vi "read_matrices.vi"() -> (0 "Matrix Matlab":T1, 1 "Trajectory":T1)   [LabVIEW 2021]
uses:
  <vilib>/Analysis/Matrix/Datatypes/RealMatrix.ctl
  <vilib>/Utility/file.llb/Read Delimited Spreadsheet (DBL).vi
  <vilib>/Analysis/Matrix/NI_Matrix.lvlib
panel:
  out "error out 2":errorcluster
  in  "delimiter (,) 2":string=","
  in  "error in (no error) 2":errorcluster
  in  "file path (dialog if empty) 2":path=path "c:/ni-rt/startup/trajectorymat.csv"
  out "error out":errorcluster
  in  "delimiter (,)":string=","
  in  "error in (no error)":errorcluster
  in  "file path (dialog if empty)":path=path "c:/ni-rt/startup/matrixmat.csv"
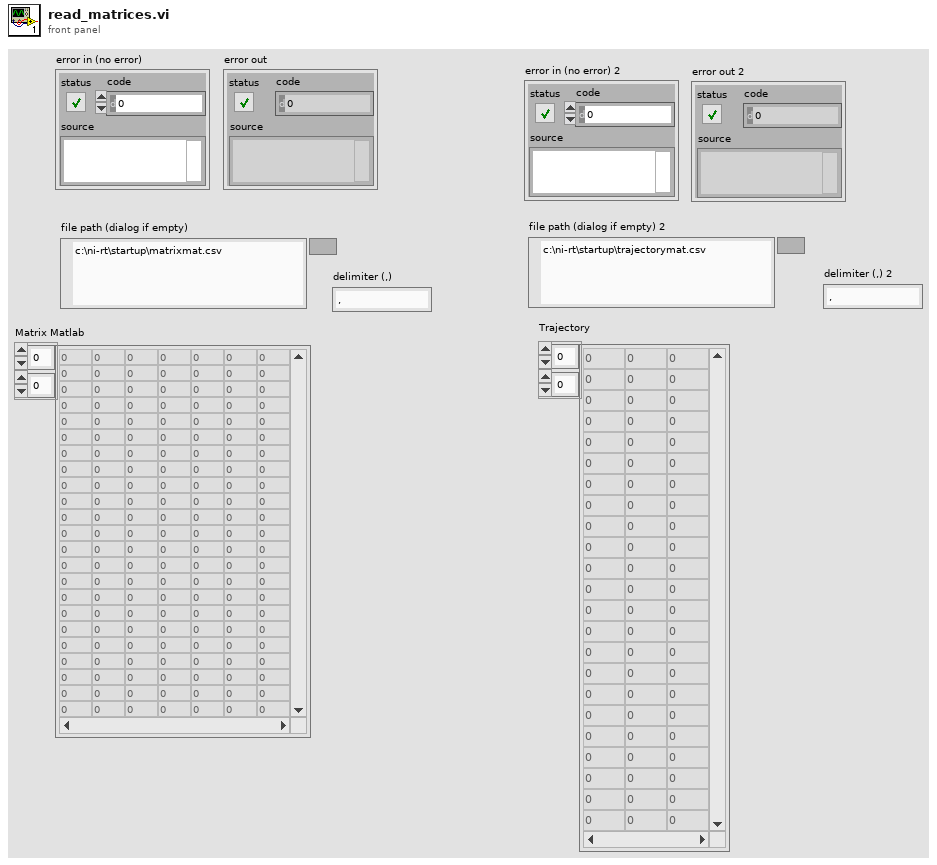
[diagram p1: front panel]
types:
  T1 = typedef "NI_Matrix.lvlib/RealMatrix.ctl" = dbl[][]
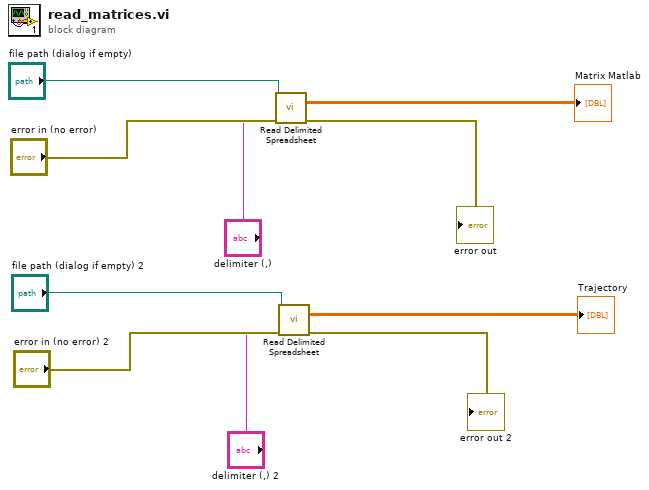
[diagram p0: block diagram]
diagram:
  n1 = call-poly <vilib>:"Read Delimited Spreadsheet.vi"("file path (dialog if empty)"="file path (dialog if empty)", "error in (no error)"="error in (no error)", "delimiter (\\t)"="delimiter (,)") -> ("all rows"=→"Matrix Matlab":dbl[][], "error out"=→"error out":errorcluster)  [unwired: 7 in, 4 out]
  n2 = call-poly <vilib>:"Read Delimited Spreadsheet.vi"("file path (dialog if empty)"="file path (dialog if empty) 2", "error in (no error)"="error in (no error) 2", "delimiter (\\t)"="delimiter (,) 2") -> ("all rows"=→"Trajectory":dbl[][], "error out"=→"error out 2":errorcluster)  [unwired: 7 in, 4 out]
